vi "sterowanie kartezjasnkie.vi"(0 "p":dbl, 5 "L":dbl, 7 "Pz":dbl(slide) scale=0.0..1149.0, 9 "Py":dbl(slide) scale=0.0..1075.0, 11 "Px":dbl(slide) scale=0.0..1075.0) -> (4 "q1":dbl format="%.2f", 6 "q2":dbl format="%.2f", 8 "q3":dbl format="%.2f", 10 "q4":dbl format="%.2f", 15 "q5":dbl format="%.2f")   [LabVIEW 2015]
panel:
  out "Pcz":i32
  out "Pcy":i32
  out "Pcx":i32
  out "k":i32
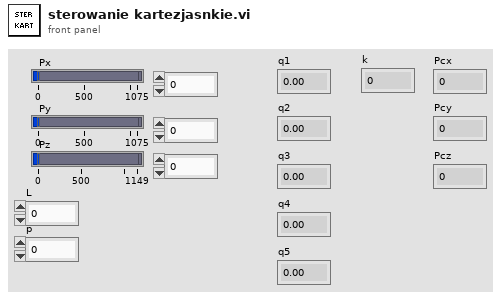
[diagram p1: front panel]
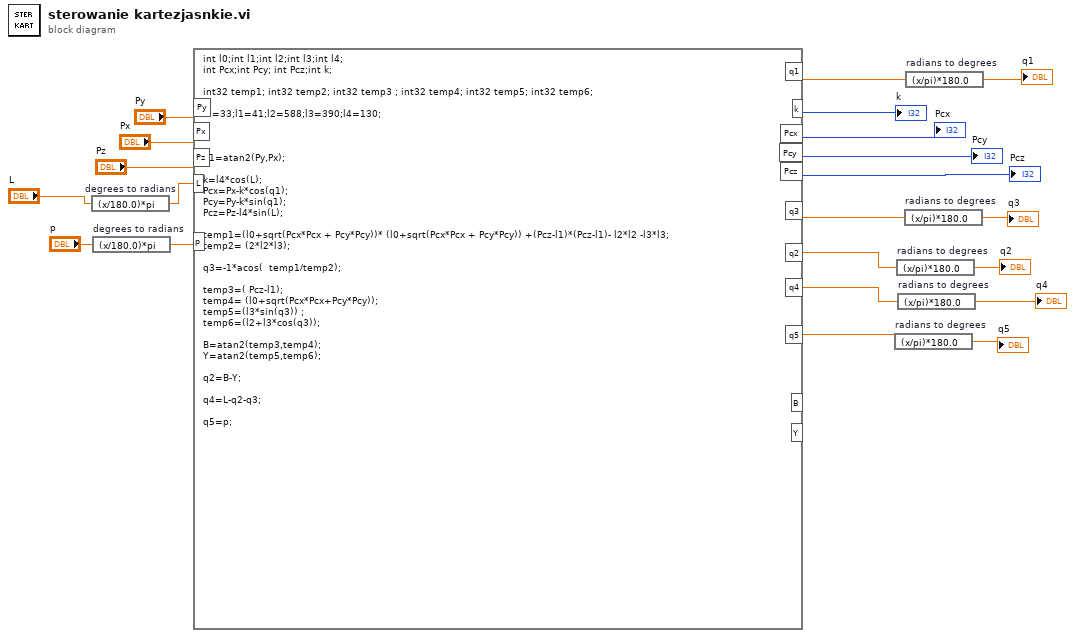
[diagram p0: block diagram]
diagram:
  n1 = expression code="(x/180.0)*pi" "degrees to radians"("L") -> (w9:dbl)
  n2 = expression code="(x/180.0)*pi" "degrees to radians"("p") -> (w2:dbl)
  n3 = formula code="int l0;int l1;int l2;int l3;int l4; \nint Pcx;int Pcy; int Pcz;int k;\n\nint32 temp1; int32 temp2; int32 temp3 ; int32 temp4; int32 temp5; int32 temp6;\n\nl0=33;l1=41;l2=588;l3=390;l4=130;\n\n\n\nq1=atan2(Py,Px); \n\nk=l4*cos(L);\nPcx=Px-k*cos(q1);\nPcy=Py-k*sin(q1);\nPcz=Pz-l4*sin(L);\n\ntemp1=(l0+sqrt(Pcx*Pcx + Pcy*Pcy))* (l0+sqrt(Pcx*Pcx + Pcy*Pcy)) +(Pcz-l1)*(Pcz-l1)- l2*l2 -l3*l3;\ntemp2= (2*l2*l3);\n\nq3=-1*acos(  temp1/temp2);\n\ntemp3=( Pcz-l1);\ntemp4= (l0+sqrt(Pcx*Pcx+Pcy*Pcy));\ntemp5=(l3*sin(q3)) ;\ntemp6=(l2+l3*cos(q3));\n\nB=atan2(temp3,temp4);\nY=atan2(temp5,temp6);\n\nq2=B-Y;\n\nq4=L-q2-q3;\n\nq5=p;"("Py"="Py", "Px"="Px", "Pz"="Pz", "L"=w9, "p"=w2) -> ("q1"=w19:dbl, "Pcx"=→"Pcx":i32, "Pcy"=→"Pcy":i32, "Pcz"=→"Pcz":i32, "k"=→"k":i32, "q3"=w12:dbl, "q2"=w8:dbl, "q4"=w6:dbl, "q5"=w4:dbl)  [unwired: 2 out]
  n4 = expression code="(x/pi)*180.0" "radians to degrees"(w4) -> (→"q5":dbl)
  n5 = expression code="(x/pi)*180.0" "radians to degrees"(w8) -> (→"q2":dbl)
  n6 = expression code="(x/pi)*180.0" "radians to degrees"(w6) -> (→"q4":dbl)
  n7 = expression code="(x/pi)*180.0" "radians to degrees"(w12) -> (→"q3":dbl)
  n8 = expression code="(x/pi)*180.0" "radians to degrees"(w19) -> (→"q1":dbl)
